vi "Data_Adquisition.vi"(6 "error in":errorcluster, 8 "Mean Iterations":i32, 9 "task in":refnum<k21>) -> (0 "error out":errorcluster, 1 "Sample taken":bool, 2 "mean and std":cluster{"mean":dbl, "standard deviation":dbl}, 3 "task out":refnum<k21>)   [LabVIEW 2024]
uses:
  <vilib>/DAQmx/read.llb/DAQmx Read (Analog DBL 1Chan 1Samp).vi
  <vilib>/DAQmx/miscellaneous.llb/DAQmx Fill In Error Info.vi
  <vilib>/Analysis/NI_AALBase.lvlib
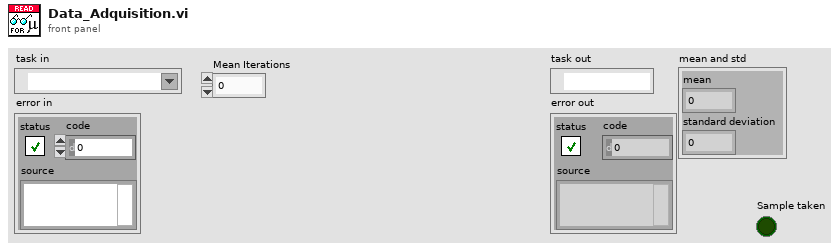
[diagram p1: front panel]
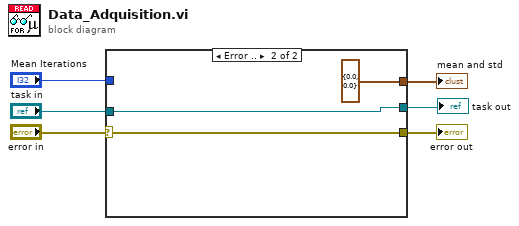
[diagram p0: block diagram]
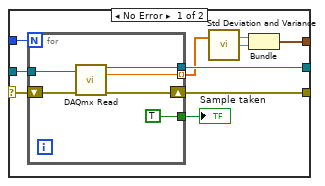
[diagram p2: hidden frame]
diagram:
  n1 = case shown="Error .." "error in" {
    selector: "error in" -> [w7 w25]
    tunnel: [w16 w24] -> w6
    tunnel: "task in" -> [w15 w24]
    tunnel: [w14 w25] -> w4
    tunnel: "Mean Iterations" -> [w12 _]
    tunnel: [w9 cluster{"mean":dbl, "standard deviation":dbl} {"mean"=0.0, "standard deviation"=0.0}] -> w2
    frame No Error {
      n2 = for {
        N: w12 -> [_]
        tunnel: [w22] -> w16
        tunnel: w15 -> [w21]
        shift-right: [w20] -> w14
        shift-left: w7 -> [w19]
        tunnel: [w18] -> w13 mode=indexing
        tunnel: [TRUE] -> w8
        n3 = call-poly <vilib>:"DAQmx Read.vi"("task/channels in"=w21, "error in"=w19) -> ("task out"=w22:refnum<k21>, "data"=w18:dbl, "error out"=w20:errorcluster)  [unwired: 11 in]
      }
      "Sample taken" <- w8
      n4 = call <vilib>:"Std Deviation and Variance.vi"("X"=w13) -> ("mean"=w11:dbl, "standard deviation"=w10:dbl)  [unwired: 1 in, 1 out]
      n5 = Bundle("mean"=w11, "standard deviation"=w10) -> (w9:cluster{"mean":dbl, "standard deviation":dbl})  [unwired: 1 in]
    }
    frame Error {
    }
  }
  "task out" <- w6
  "error out" <- w4
  "mean and std" <- w2
